vi "Rst_Or.vi"(0 "BAR rst":bool, 5 "L/Min rst":bool, 7 "BPM rst":bool, 9 "A*C rst":bool, 11 "error In":errorcluster, 12 "RST_COLOR":refnum<vi>) -> (3 "Rst":string, 4 "BAR":bool, 6 "L/Min":bool, 8 "BPM":bool, 10 "A*C":bool, 15 "error out":errorcluster)   [LabVIEW 2017]
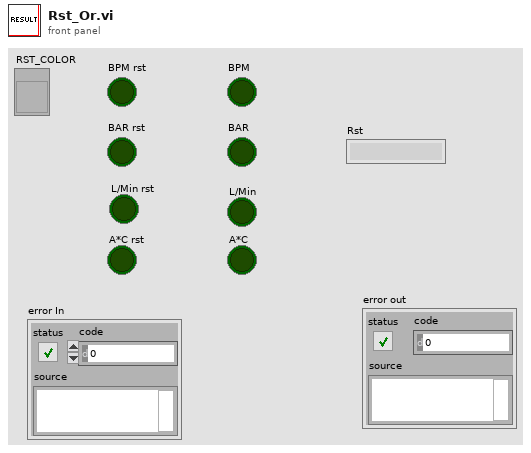
[diagram p1: front panel]
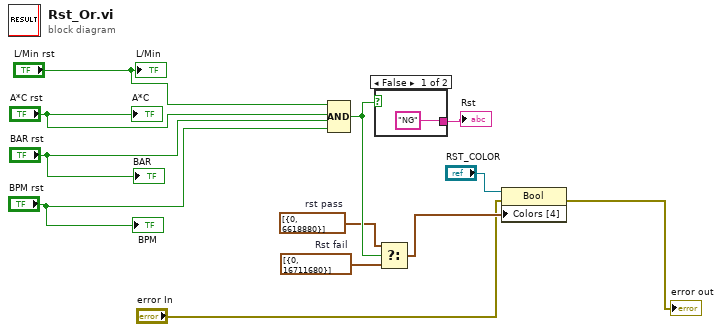
[diagram p0: block diagram]
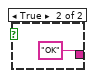
[diagram p2: hidden frame]
diagram:
  w7 = cluster{u32, u32}[] [{0, 6618880}]  # rst pass
  w6 = cluster{u32, u32}[] [{0, 16711680}]  # Rst fail
  n1 = Compound Arithmetic op=AND("L/Min rst", "A*C rst", "BAR rst", "BPM rst") -> (w12:bool)
  n2 = case shown="False" w12 {
    tunnel: ["NG" "OK"] -> w11
    frame False {
    }
    frame True {
    }
  }
  "Rst" <- w11
  n3 = Select(t=w7, s=w12, f=w6) -> (s? t:f=w4:cluster{u32, u32}[])
  n4 = property on="Property Node" class="Bool"(reference="RST_COLOR", error in="error In", "Colors [4]"=w4) -> (error out=→"error out":errorcluster)  [unwired: 1 out]
  "L/Min" <- "L/Min rst"
  "A*C" <- "A*C rst"
  "BAR" <- "BAR rst"
  "BPM" <- "BPM rst"
